vi "标签回退.vi"(8 "error in":errorcluster caption="错误输入（无错误）", 10 "标签（版本）":string, 11 "仓库路径":path=path "E:/学习文件/Git插件/test") -> (0 "error out":errorcluster caption="错误输出", 1 "standard error":string caption="标准错误", 2 "standard output":string caption="标准输出", 3 "仓库路径":path=path "E:/学习文件/Git插件/test")   [LabVIEW 2018]
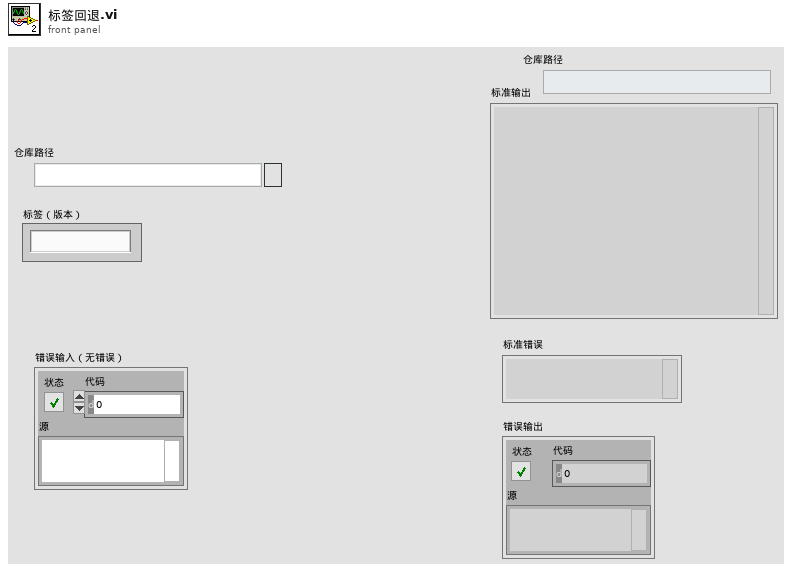
[diagram p1: front panel]
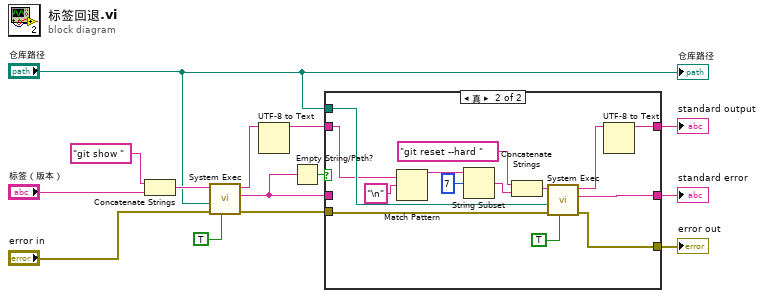
[diagram p0: block diagram]
diagram:
  n1 = Concatenate Strings("git show " ("command line"), "标签（版本）") -> (w10:string)
  n2 = call <vilib>:"System Exec.vi"("run minimized? (F)"=TRUE, "error in (no error)"="error in", "working directory"="仓库路径", "command line"=w10) -> ("error out"=w8:errorcluster, "standard error"=w2:string, "standard output"=w14:string)  [unwired: 4 in, 1 out]
  n3 = UTF-8 to Text ("UTF-8至文本转换")(11:w14) -> (3:w1:string)  [unwired: 2 in, 1 out]
  n4 = Empty String/Path?(string/path=w2) -> (empty?=w3:bool)
  n5 = case shown="真" w3 {
    tunnel: w8 -> [w16 w27]
    tunnel: "仓库路径" -> [_ w26]
    tunnel: [w16 w25] -> w6
    tunnel: [w15 w24] -> w5
    tunnel: [w17 w23] -> w4
    tunnel: w1 -> [w15 w19]
    tunnel: w2 -> [w17 _]
    frame False {
    }
    frame True {
      n6 = Match Pattern(string=w19, regular expression="\n" ("正则表达式")) -> (before substring=w22:string)  [unwired: 1 in, 3 out]
      n7 = String Subset(string=w22, offset (0)=7 ("偏移量(0)")) -> (substring=w18:string)  [unwired: 1 in]
      n8 = Concatenate Strings("git reset --hard " ("command line"), w18) -> (w30:string)
      n9 = call <vilib>:"System Exec.vi"("run minimized? (F)"=TRUE, "error in (no error)"=w27, "working directory"=w26, "command line"=w30) -> ("error out"=w25:errorcluster, "standard error"=w23:string, "standard output"=w28:string)  [unwired: 4 in, 1 out]
      n10 = UTF-8 to Text ("UTF-8至文本转换")(11:w28) -> (3:w24:string)  [unwired: 2 in, 1 out]
    }
  }
  "standard output" <- w5
  "standard error" <- w4
  "error out" <- w6
  "仓库路径" <- "仓库路径"
